vi "ClawManualOverride.vi"(7 "Claw Manual Input":dbl format="%#_13g", 10 "Claw States":T1, 11 "Claw PID Input":dbl format="%#_13g") -> (3 "Claw Output":dbl)   [LabVIEW 2014]
uses:
  Typedefs/ClawStates.ctl
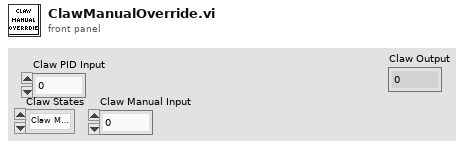
[diagram p1: front panel]
types:
  T1 = typedef "ClawStates.ctl" = enum16{"Claw Manual ", "Claw Open", "Claw Closed", "Claw Slight Open"}
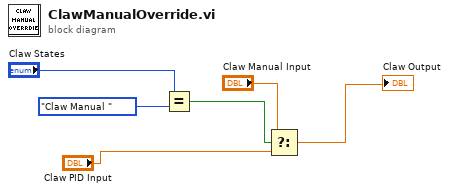
[diagram p0: block diagram]
diagram:
  n1 = Equal?(x="Claw States", y=ClawStates."Claw Manual ") -> (x = y?=w3:bool)
  n2 = Select(t="Claw Manual Input", s=w3, f="Claw PID Input") -> (s? t:f=→"Claw Output":dbl)
